vi "ChangeArray(SubVI).vi"(4 "NumPlot":dbl, 6 "element":T1 {"Color" format="%x"}, 7 "XYGraph Refnum":refnum<vi>, 8 "Error In":errorcluster, 9 "Boolean":bool, 10 "ComboBox in":refnum<vi>, 11 "LVObjectRefNum in":refnum<vi>) -> (0 "Error Out":errorcluster)   [LabVIEW 2018]
uses:
  CTL/Line.ctl
  Windows/Settings/View.ctl
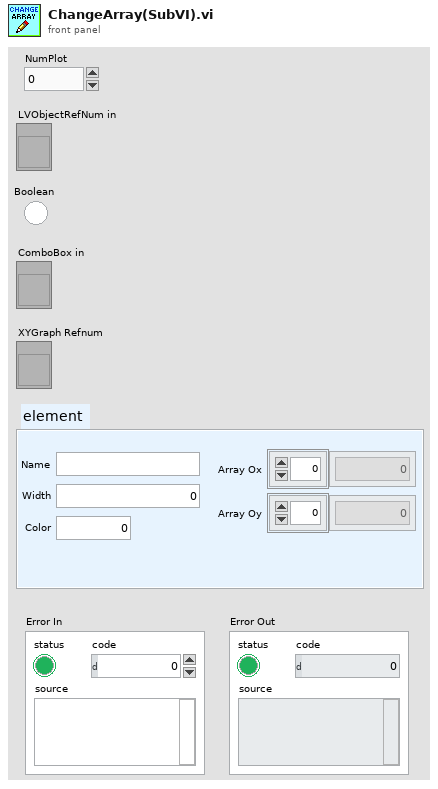
[diagram p1: front panel]
types:
  T1 = typedef "Line.ctl" = cluster{"Width":dbl, "Color":i64, "Array Oy":dbl[], "Array Ox":dbl[], "Name":string, "Plot Visible":T2}
  T2 = typedef "View.ctl" = bool
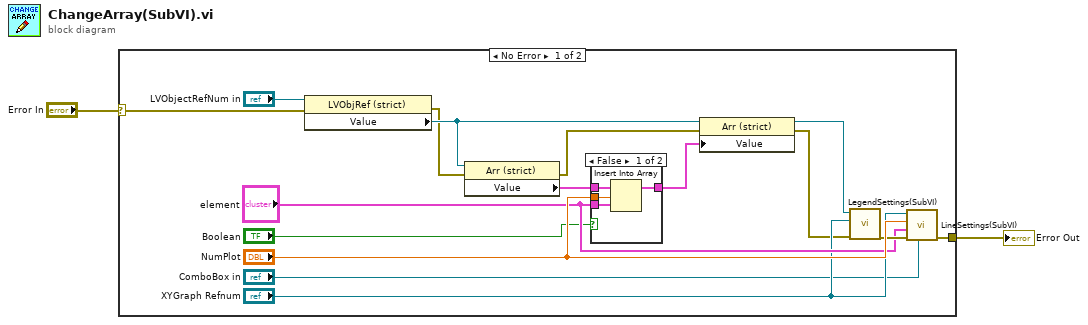
[diagram p0: block diagram]
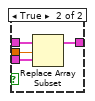
[diagram p2: hidden frame]
diagram:
  n1 = case shown="No Error" "Error In" {
    selector: "Error In" -> [w6 w27]
    tunnel: [w3 w27] -> w1
    frame No Error {
      n2 = property on="Property Node" class="LVObjRef (strict)"(reference="LVObjectRefNum in", error in=w6) -> (error out=w5:errorcluster, "Value"=w9:refnum<vi>)  [unwired: 1 out]
      n3 = property on="Property Node" class="Arr (strict)"(reference=w9, error in=w5) -> (error out=w4:errorcluster, "Value"=w8:T1[])  [unwired: 1 out]
      n4 = case shown="False" "Boolean" {
        tunnel: "NumPlot" -> [w19 w23]
        tunnel: w8 -> [w22 w26]
        tunnel: "element" -> [w20 w25]
        tunnel: [w21 w24] -> w10
        frame False {
          n5 = Insert Into Array(array=w22, index=w19, new element=w20) -> (w21:T1[])
        }
        frame True {
          n6 = Replace Array Subset(array=w26, new element=w25, index=w23) -> (w24:T1[])
        }
      }
      n7 = property on="Property Node" class="Arr (strict)"(reference=w9, error in=w4, "Value"=w10) -> (reference out=w13:refnum<vi>, error out=w14:errorcluster)
      n8 = call "LegendSettings(SubVI).vi"("Error In"=w14, "XYGraph Refnum"="XYGraph Refnum", "Arr Refnum"=w13) -> ("Error Out"=w17:errorcluster)  [unwired: 8 in]
      n9 = call "LineSettings(SubVI).vi"("LVObjRef Refnum"="ComboBox in", "Error In"=w17, "element"="element", "NumPlot"="NumPlot", "XYGraph in"="XYGraph Refnum") -> ("Error Out"=w3:errorcluster)  [unwired: 6 in]
    }
    frame Error {
    }
  }
  "Error Out" <- w1
